vi "New Message.vi"(8 "error in (no error)":errorcluster, 9 "New Message":string, 10 "From":string, 11 "Chat Window Model in":refnum<class "Chat Window Model.lvclass">) -> (0 "error out":errorcluster, 3 "Chat Window Model out":refnum<class "Chat Window Model.lvclass">)   [LabVIEW 2020, in "Chat Window Model.lvlib" / "Chat Window Model.lvclass"]
uses:
  Chat Window Model.lvclass
  Chat Window Model.lvclass/Chat Window Model.ctl
  Chat Window UI Controller/Chat Window UI Controller Messages/Update Message Window Msg/Update Message Window Msg.lvclass/Update Message Window Msg.ctl
  <vilib>/ActorFramework/Message Enqueuer/Message Enqueuer.lvclass/Message Enqueuer.ctl
  <vilib>/ActorFramework/Message Enqueuer/Enqueue.vi
  Chat Window UI Controller/Chat Window UI Controller Messages/Update Message Window Msg/Update Message Window Msg.lvclass
  C:/Program Files/National Instruments/LabVIEW 2020/vi.lib/ActorFramework/Message/Message.lvclass
  <vilib>/ActorFramework/Message Priority Queue/Priority Enqueue.vi
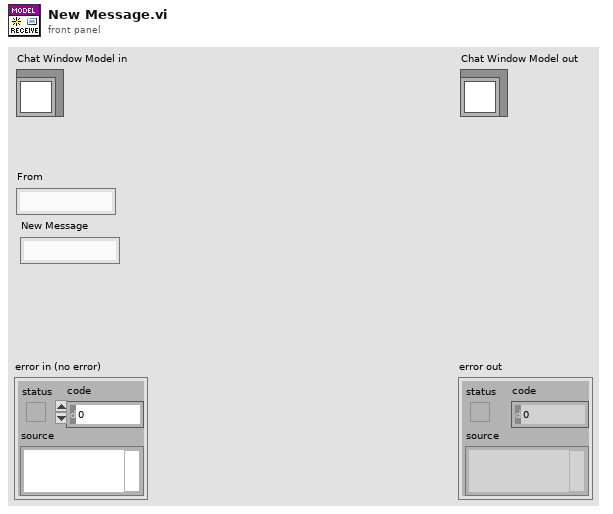
[diagram p1: front panel]
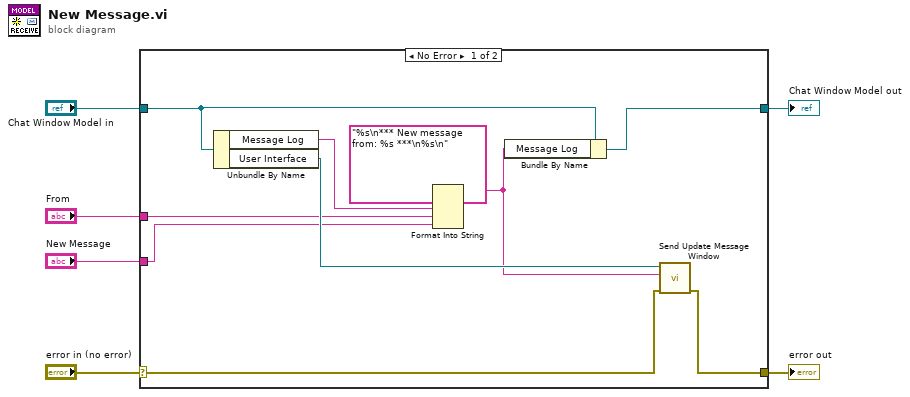
[diagram p0: block diagram]
diagram:
  n1 = case shown="No Error" "error in (no error)" {
    selector: "error in (no error)" -> [w13 w18]
    tunnel: [w12 w18] -> w5
    tunnel: [w15 w17] -> w3
    tunnel: "Chat Window Model in" -> [w16 w17]
    tunnel: "New Message" -> [w8 _]
    tunnel: "From" -> [w9 _]
    frame No Error {
      n2 = Unbundle By Name(w16) -> ("Message Log"=w10:string, "User Interface"=w14:refnum<class "Message Enqueuer.lvclass">)
      n3 = Format Into String(format string="%s\n*** New message from: %s ***\n%s\n", w10, w9, w8) -> (resulting string=w7:string)  [unwired: 2 in, 1 out]
      n4 = Bundle By Name(cluster=w16, "Message Log"=w7) -> (w15:refnum<class "Chat Window Model.lvclass">)
      n5 = call "Send Update Message Window.vi"("error in (no error)"=w13, "Message"=w7, "Message Enqueuer"=w14) -> ("error out"=w12:errorcluster)  [unwired: 7 in, 1 out]
    }
    frame Error {
    }
  }
  "error out" <- w5
  "Chat Window Model out" <- w3
